vi "Key Logging.vi"() -> ()   [LabVIEW 2012]
panel:
  out "Log Error":errorcluster
  in  "stop":bool
  in  "Save":bool caption="3) After scanning... click this to save the log."
  in  "Scan":string caption="2) Scan barcode into here"
  in  "Folder":path caption="1) Select a Folder to Save Logs To"
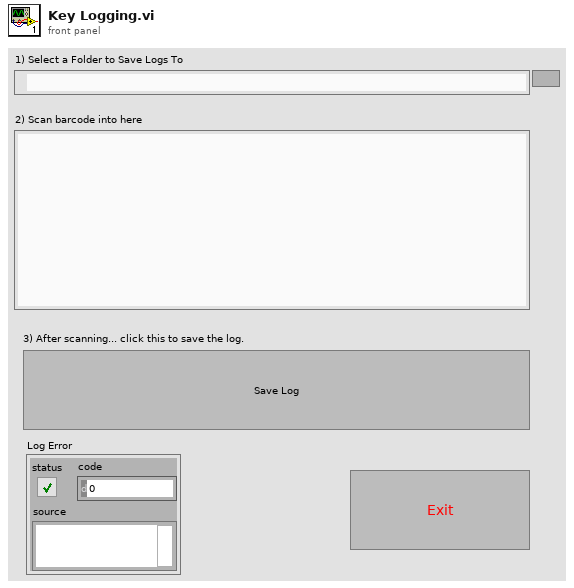
[diagram p1: front panel]
types:
  T1 = enum16{"open", "replace", "create", "open or create", "replace or create", "replace or create with confirmation"}
  T2 = typedef "eventvkey.ctl" = enum16{"ASCII", "Enter", "Return", "Shift", "Ctrl", "Alt", "Cmd", "Opt", "Caps", "NumLock", "Clear", "Break", "Up", "Down", "Left", "Right", "Insert", "Delete", "Home", "End", "PageUp", "PageDown", "Escape", "Help", "Pause", "ScrollLock", "F1", "F2", "F3", "F4", "F5", "F6", "F7", "F8", "F9", "F10", "F11", "F12", "F13", "F14", "F15", "F16", "F17", "F18", "F19", "F20", "F21", "F22", "F23", "F24", "Play", "VolumeUp", "VolumeDown", "Mute", "Two Byte Char"}
  T3 = cluster{"Shift":bool, "Ctrl":bool, "Alt":bool, "Cmd":bool, "Opt":bool}
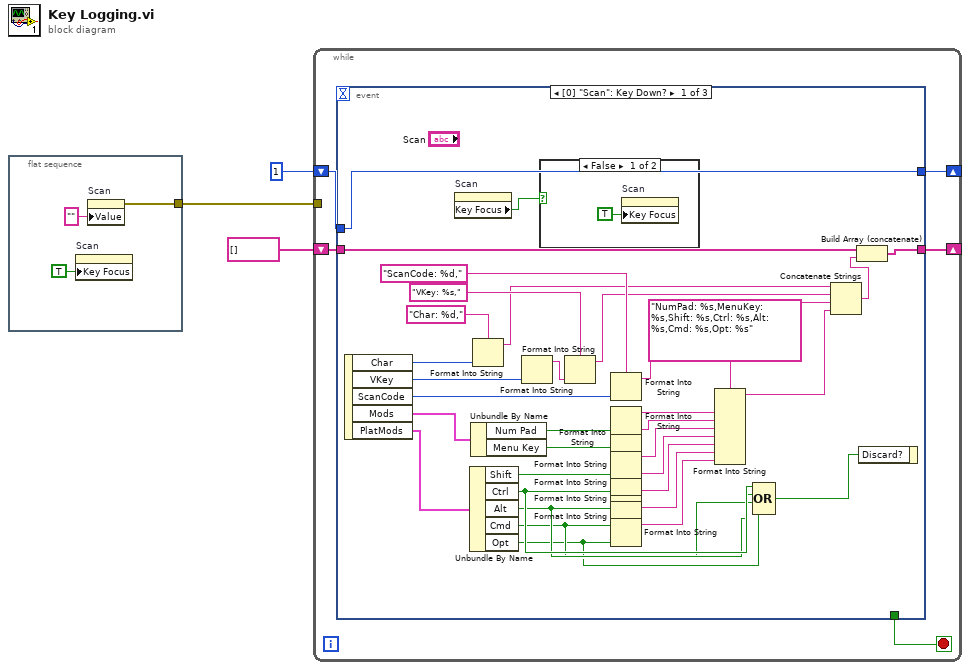
[diagram p0: block diagram]
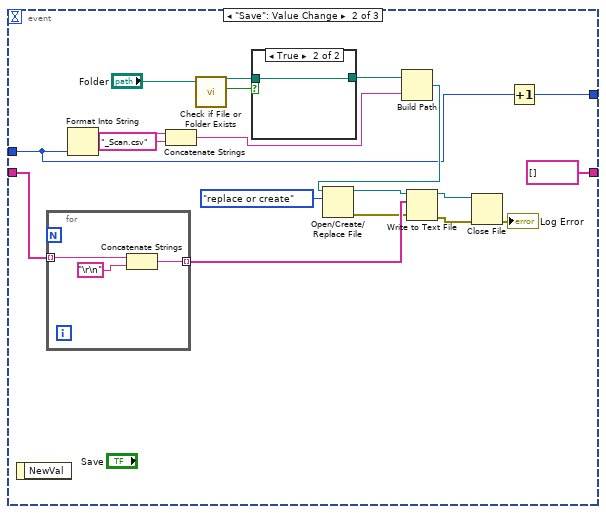
[diagram p3: hidden frame]
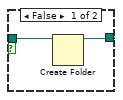
[diagram p4: hidden frame]
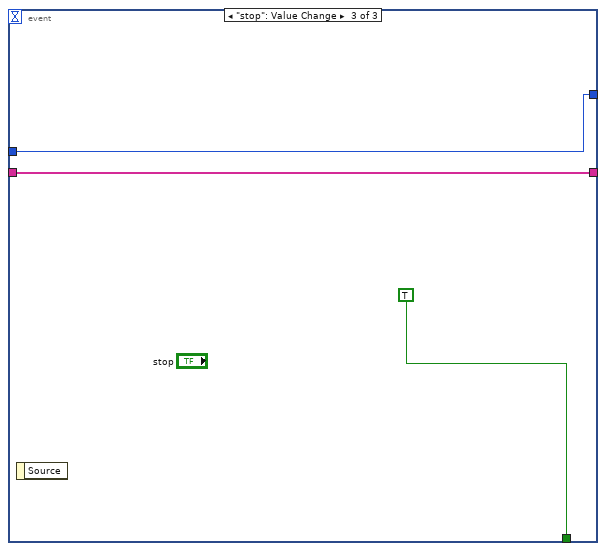
[diagram p5: hidden frame]
diagram:
  n1 = flat-sequence {
    tunnel: [w5] -> w3
    frame #0 {
      n2 = property on="Scan" class="Str"("Key Focus"=TRUE) -> ()  [unwired: 2 in, 2 out]
      n3 = property on="Scan" class="Str"("Value"="" ("Scan")) -> (error out=w5:errorcluster)  [unwired: 2 in, 1 out]
    }
  }
  n4 = while {
    tunnel: w3 -> [_]
    shift-right: [w9] -> _
    shift-left: string[] [] ("output cluster") -> [w11]
    shift-right: [w7] -> _
    shift-left: 1 -> [w8]
    stop <- w10 stop-if-true
    n5 = event shown="[0] \"Scan\": Key Down?" {
      selector: _ -> [_ _ _]
      dyn-events: _ -> [_ _ _]
      timeout: _ -> [_ _ _]
      tunnel: w11 -> [w45 w64 w73]
      tunnel: [w44 string[] [] w73] -> w9
      tunnel: [_ _ TRUE] -> w10
      tunnel: w8 -> [w18 w48 w72]
      tunnel: [w18 w47 w72] -> w7
      event "Scan": Key Down? {
        n6 = event-data() -> ("Char"=w43:i16, "VKey"=w39:T2, "ScanCode"=w42:i16, "Mods"=w36:cluster{"Num Pad":bool, "Menu Key":bool}, "PlatMods"=w35:T3)  [unwired: 1 in]
        n7 = property on="Scan" class="Str"() -> ("Key Focus"=w12:bool)  [unwired: 2 in, 2 out]
        n8 = Unbundle By Name(w35) -> ("Shift"=w32:bool, "Ctrl"=w17:bool, "Alt"=w16:bool, "Cmd"=w15:bool, "Opt"=w14:bool)
        n9 = Unbundle By Name(w36) -> ("Num Pad"=w34:bool, "Menu Key"=w33:bool)
        n10 = Format Into String(format string="Char: %d,", w43) -> (resulting string=w23:string)  [unwired: 2 in, 1 out]
        n11 = Format Into String(w39) -> (resulting string=w38:string)  [unwired: 3 in, 1 out]
        n12 = case shown="False" w12 {
          frame False {
            n13 = property on="Scan" class="Str"("Key Focus"=TRUE) -> ()  [unwired: 2 in, 2 out]
          }
          frame True {
          }
        }
        n14 = Format Into String(format string="VKey: %s,", w38) -> (resulting string=w22:string)  [unwired: 2 in, 1 out]
        n15 = Format Into String(format string="ScanCode: %d,", w42) -> (resulting string=w21:string)  [unwired: 2 in, 1 out]
        n16 = Format Into String(w34) -> (resulting string=w30:string)  [unwired: 3 in, 1 out]
        n17 = Format Into String(w33) -> (resulting string=w29:string)  [unwired: 3 in, 1 out]
        n18 = Format Into String(w32) -> (resulting string=w28:string)  [unwired: 3 in, 1 out]
        n19 = Format Into String(w17) -> (resulting string=w27:string)  [unwired: 3 in, 1 out]
        n20 = Format Into String(w16) -> (resulting string=w26:string)  [unwired: 3 in, 1 out]
        n21 = Format Into String(w15) -> (resulting string=w25:string)  [unwired: 3 in, 1 out]
        n22 = Format Into String(w14) -> (resulting string=w24:string)  [unwired: 3 in, 1 out]
        n23 = Format Into String(format string="NumPad: %s,MenuKey: %s,Shift: %s,Ctrl: %s,Alt: %s,Cmd: %s,Opt: %s", w30, w29, w28, w27, w26, w25, w24) -> (resulting string=w20:string)  [unwired: 2 in, 1 out]
        n24 = Compound Arithmetic op=OR(w17, w16, w15, w14) -> (w13:bool)
        n25 = Concatenate Strings(w23, w22, w21, w20) -> (w19:string)
        n26 = Build Array (concatenate)(w45, w19) -> (w44:string[])
        n27 = event-data("Discard?"=w13) -> ()  [unwired: 1 in, 1 out]
      }
      event "Save": Value Change {
        n28 = event-data() -> ()  [unwired: 1 in, 1 out]
        n29 = for {
          tunnel: w64 -> [w71] mode=indexing
          tunnel: [w69] -> w53 mode=indexing
          n30 = Concatenate Strings(w71, "\r\n") -> (w69:string)
        }
        n31 = Format Into String(w48) -> (resulting string=w59:string)  [unwired: 3 in, 1 out]
        n32 = Concatenate Strings(w59, "_Scan.csv" ("string")) -> (w57:string)
        n33 = call <vilib>:"Check if File or Folder Exists.vi"("path"="Folder") -> ("file or folder exists?"=w62:bool, "dup path"=w61:path)  [unwired: 8 in, 1 out]
        n34 = case shown="True" w62 {
          tunnel: w61 -> [w67 w68]
          tunnel: [w66 w68] -> w60
          frame False {
            n35 = Create Folder(path (use dialog)=w67) -> (created path=w66:path)  [unwired: 2 in, 2 out]
          }
          frame True {
          }
        }
        n36 = Build Path(base path=w60, name or relative path=w57) -> (appended path=w56:path)
        n37 = Open/Create/Replace File(file path (use dialog)=w56, operation (0:open)=T1."replace or create") -> (refnum out=w54:refnum<file>, error out=w50:errorcluster)  [unwired: 4 in, 1 out]
        n38 = Write to Text File(file (use dialog)=w54, text=w53, error in=w50) -> (refnum out=w51:refnum<file>, error out=w52:errorcluster)  [unwired: 1 in, 1 out]
        n39 = Close File(refnum=w51, error in=w52) -> (error out=→"Log Error":errorcluster)  [unwired: 1 out]
        n40 = Increment(x=w48) -> (x+1=w47:i32)
      }
      event "stop": Value Change {
        n41 = event-data() -> ()  [unwired: 1 in, 1 out]
      }
    }
  }
